vi "Open NIVS TDMS log.vi"(8 "error in (no error)":errorcluster, 10 "TDMS File":path) -> (0 "error out":errorcluster, 1 "Log Name":string, 2 "Sys Channel Names":string[](array[string]), 3 "tdms file out":refnum<k34>, 4 "group names":string[](array[string]), 5 "Logging Rate":dbl, 7 "Date Created":timestamp, 11 "Datapoints":u32)   [LabVIEW 2010, in "TDMS to ASCII Convert.lvlib"]
uses:
  TDMS to ASCII Convert.lvlib
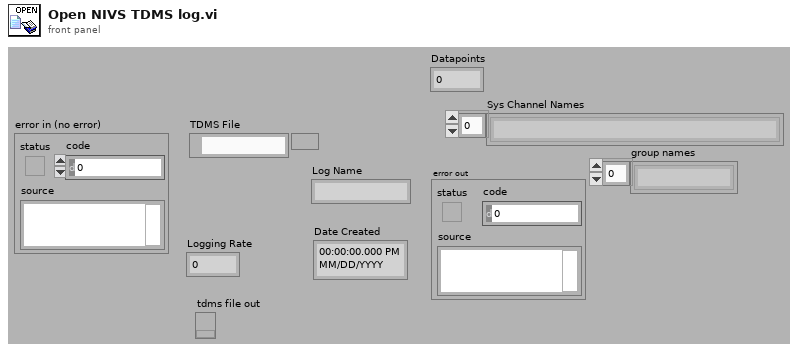
[diagram p1: front panel]
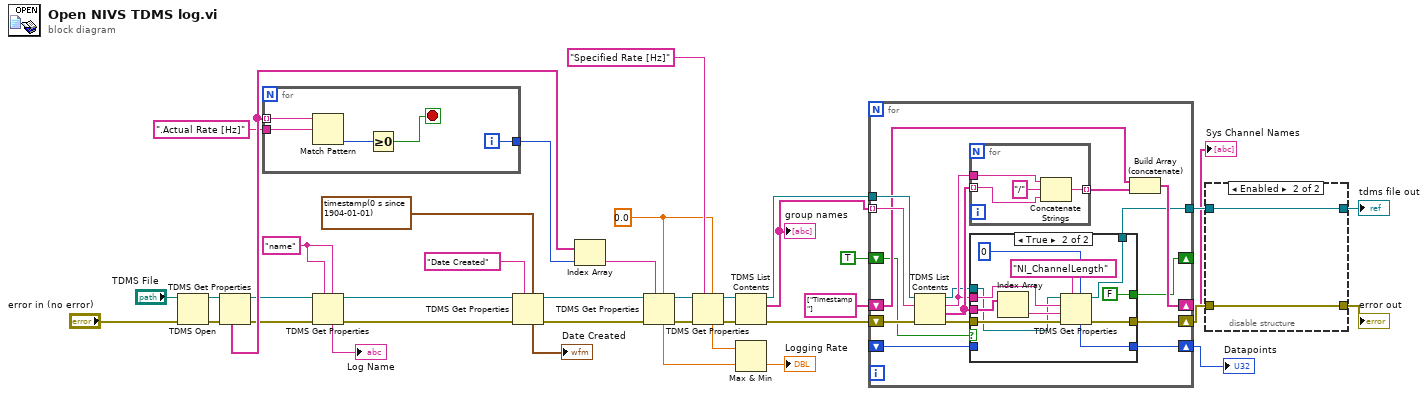
[diagram p0: block diagram]
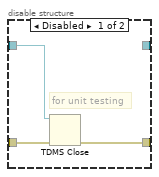
[diagram p3: hidden frame]
diagram:
  w26 = 0.0
  w14 = "name" ("property name")
  n1 = TDMS Open(8:"error in (no error)", 11:"TDMS File") -> (0:w34:errorcluster, 3:w32:refnum<k34>)  [unwired: 4 in]
  n2 = TDMS Get Properties(8:w34, 11:w32) -> (0:w35:errorcluster, 3:w33:refnum<k34>, 6:w37:string[])  [unwired: 4 in, 3 out]
  n3 = for {
    tunnel: w37 -> [w44] mode=indexing
    tunnel: ".Actual Rate [Hz]" ("regular expression") -> [w43]
    tunnel: [w40] -> w38
    i -> [w40]
    stop <- w41 stop-if-true
    n4 = Match Pattern(string=w44, regular expression=w43) -> (offset past match=w42:i32)  [unwired: 1 in, 3 out]
    n5 = Greater Or Equal To 0?(x=w42) -> (x >= 0?=w41:bool)
  }
  n6 = TDMS Get Properties(5:w14, 7:w14, 8:w35, 11:w33) -> (0:w15:errorcluster, 3:w17:refnum<k34>, 4:→"Log Name":string)  [unwired: 2 in, 3 out]
  n7 = TDMS Get Properties(5:timestamp(0 s since 1904-01-01), 7:"Date Created" ("property name"), 8:w15, 11:w17) -> (0:w16:errorcluster, 3:w18:refnum<k34>, 4:→"Date Created":timestamp)  [unwired: 2 in, 3 out]
  n8 = Index Array(array=w37, index=w38) -> (element=w39:string)
  n9 = TDMS Get Properties(5:w26, 7:w39, 8:w16, 11:w18) -> (0:w23:errorcluster, 3:w24:refnum<k34>, 4:w28:dbl)  [unwired: 2 in, 3 out]
  n10 = TDMS Get Properties(5:w26, 7:"Specified Rate [Hz]" ("property name"), 8:w23, 11:w24) -> (0:w31:errorcluster, 3:w25:refnum<k34>, 4:w29:dbl)  [unwired: 2 in, 3 out]
  n11 = TDMS List Contents(4:w31, 7:w25) -> (0:w8:errorcluster, 2:w9:string[], 3:w6:refnum<k34>)  [unwired: 1 in, 1 out]
  "group names" <- w9
  n12 = Max & Min(x=w29, y=w28) -> (min(x,y)=→"Logging Rate":dbl)  [unwired: 1 out]
  n13 = for {
    tunnel: w9 -> [w58] mode=indexing
    shift-right: [w50] -> w7
    shift-left: w8 -> [w60]
    tunnel: w6 -> [w59]
    tunnel: [w45] -> w5
    shift-right: [w55] -> w3
    shift-left: string[] ["Timestamp"] -> [w57]
    shift-right: [w49] -> _
    shift-left: TRUE -> [w54]
    shift-right: [w48] -> w1
    shift-left: _ -> [w47]
    n14 = TDMS List Contents(4:w60, 6:w58, 7:w59) -> (0:w51:errorcluster, 1:w53:string[], 2:w52:string, 3:w46:refnum<k34>)
    n15 = for {
      tunnel: w53 -> [w77] mode=indexing
      tunnel: w52 -> [w78]
      tunnel: [w76] -> w56 mode=indexing
      n16 = Concatenate Strings(w78, "/" ("string"), w77) -> (w76:string)
    }
    n17 = case shown="True" w54 {
      selector: w54 -> [w64 _]
      tunnel: w53 -> [_ w75]
      tunnel: w52 -> [_ w73]
      tunnel: w51 -> [w63 w72]
      tunnel: [w63 w71] -> w50
      tunnel: [w64 FALSE] -> w49
      tunnel: [w62 w67] -> w48
      tunnel: w47 -> [w62 _]
      tunnel: w46 -> [w61 w66]
      tunnel: [w61 w65] -> w45
      frame False {
      }
      frame True {
        n18 = Index Array(array=w75) -> (element=w74:string)  [unwired: 1 in]
        n19 = TDMS Get Properties(5:u32 0, 7:"NI_ChannelLength" ("property name"), 8:w72, 9:w74, 10:w73, 11:w66) -> (0:w71:errorcluster, 3:w65:refnum<k34>, 4:w67:u32)  [unwired: 3 out]
      }
    }
    n20 = Build Array (concatenate)(w57, w56) -> (w55:string[])
  }
  "Sys Channel Names" <- w3
  "Datapoints" <- w1
  n21 = disable-structure shown="Enabled" {
    disable-tunnel: w7 -> [w81 w83]
    disable-tunnel: [w82 w83] -> w11
    disable-tunnel: w5 -> [w80 w84]
    disable-tunnel: [_ w84] -> w10
    frame Disabled {
      # "for unit testing"
      n22 = TDMS Close(8:w81, 11:w80) -> (0:w82:errorcluster)  [unwired: 1 out]
    }
    frame Enabled {
    }
  }
  "tdms file out" <- w10
  "error out" <- w11
